vi "Main.vi"(8 "error in":errorcluster, 11 "Main View in":refnum<class "Main View.lvclass">) -> (0 "error out":errorcluster, 3 "Main View out":refnum<class "Main View.lvclass">)   [LabVIEW 2018, in "Main View.lvclass"]
doc: "The Queued Message Handler of a Worker."
uses:
  Main View.lvclass
  D:/Program Files (x86)/National Instruments/LabVIEW 2018/vi.lib/addons/_Workers/Library/Classes/Worker/Worker.lvclass
  Menu Button.ctl
  Main View.lvclass/Main View.ctl
  <vilib>/addons/_Workers/Library/Classes/Worker/Worker.lvclass/Worker.ctl
  Aging View/Aging View.lvclass
  Query Data/Query Data.lvclass
  About View/About View.lvclass
  Settings View/Settings View.lvclass
  <vilib>/addons/_Workers/Library/Classes/Message/Enqueue Message to Queue.vi
  <vilib>/addons/_Workers/Library/Classes/Message/Enqueue Message to Self v2.vi
  Acquire Data/Acquire Data.lvclass
  Save Data/Save Data.lvclass
  Initialization Data.ctl
  <vilib>/addons/_Workers/Library/Classes/Worker/Worker.lvclass
  <vilib>/addons/_Workers/Library/Classes/Message/Message.lvclass
  D:/Program Files (x86)/National Instruments/LabVIEW 2018/vi.lib/addons/_Workers/Library/Classes/Workers Object/Workers Object.lvclass
panel:
  in  "Menu Button":T1
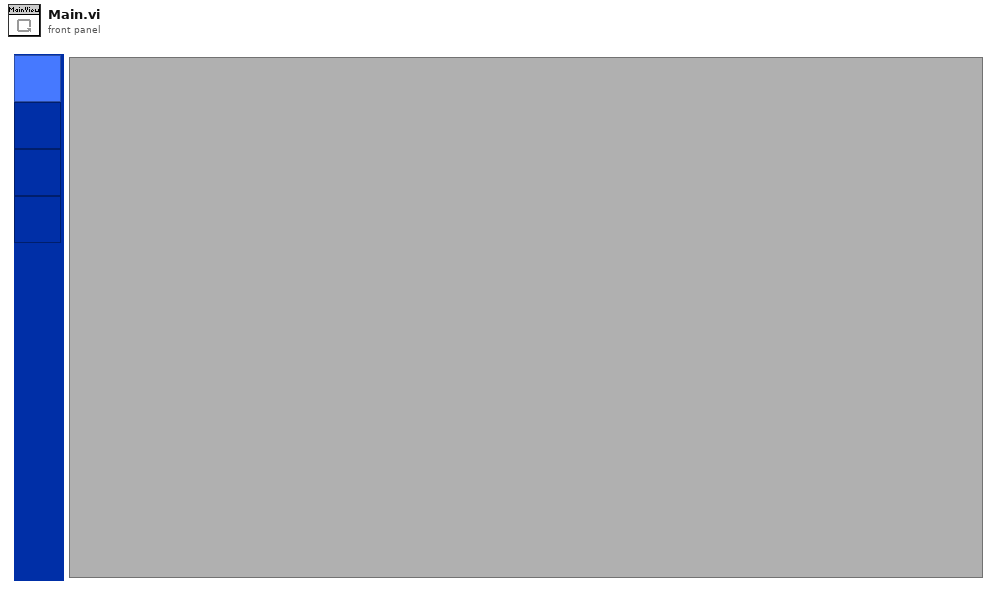
[diagram p1: front panel]
types:
  T1 = typedef "Main View.lvclass/Menu Button.ctl" = enum32{"Settings Button", "Aging Button", "Query Button", "Help Button"}
  T2 = typedef "Main View.lvclass/Initialization Data.ctl" = cluster{}
  T3 = typedef "Workers.lvlib/Case Label.ctl" = string
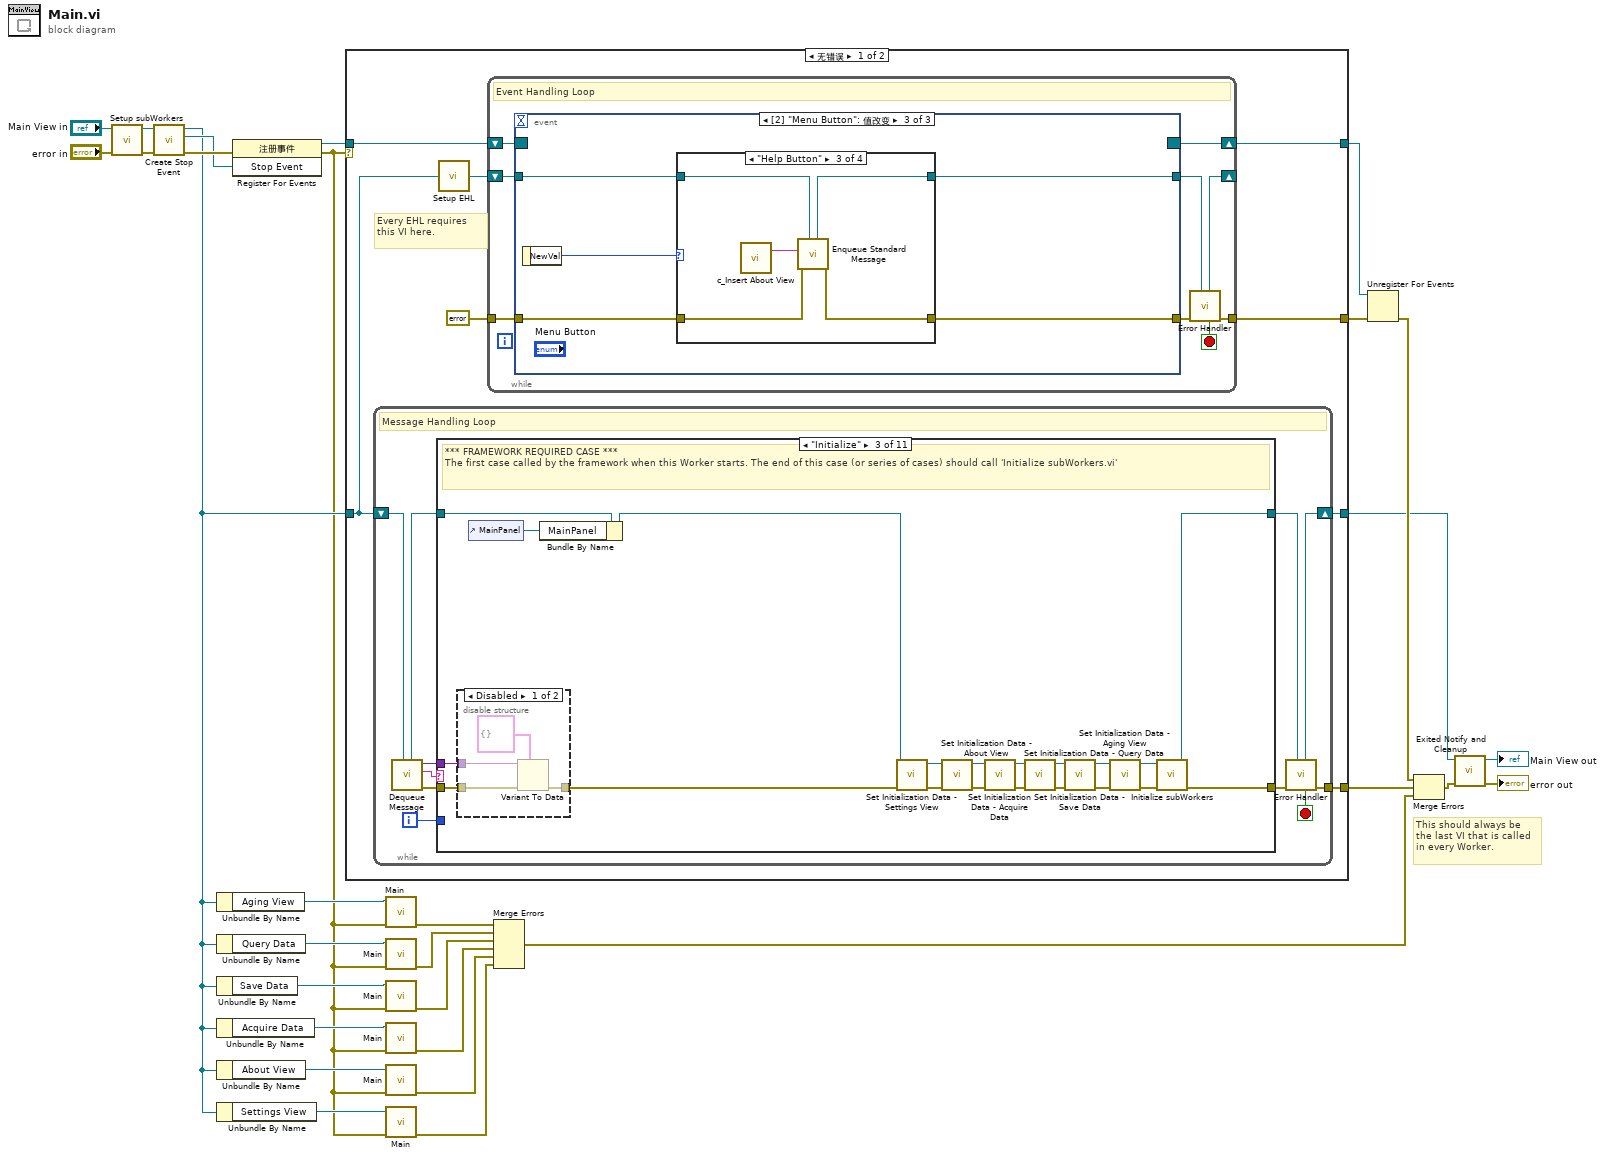
[diagram p0: block diagram]
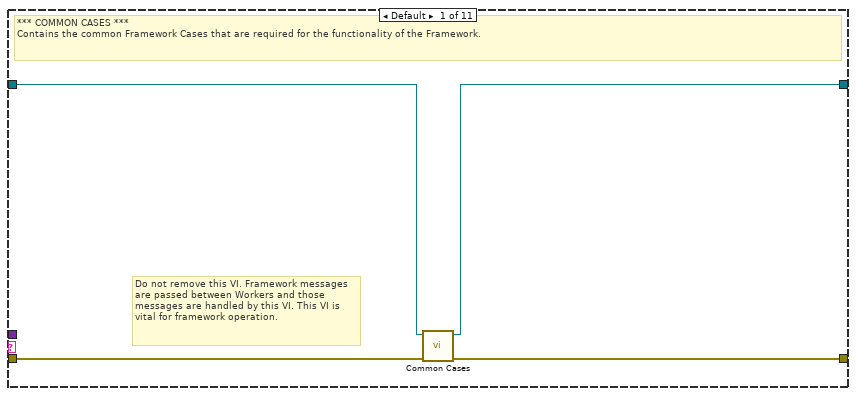
[diagram p2: hidden frame]
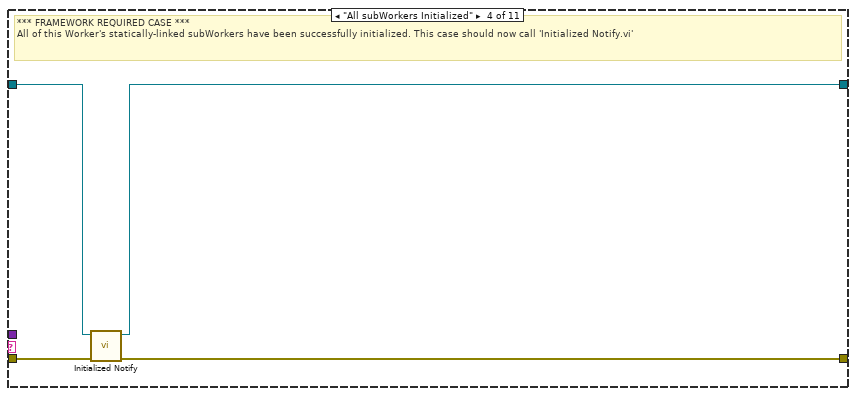
[diagram p5: hidden frame]
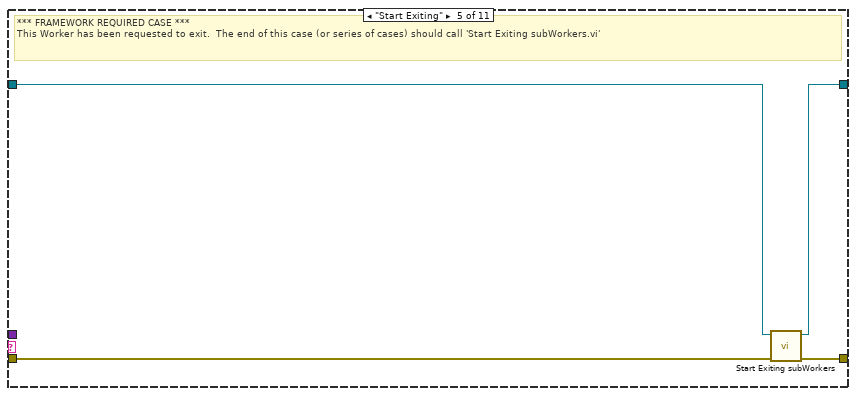
[diagram p6: hidden frame]
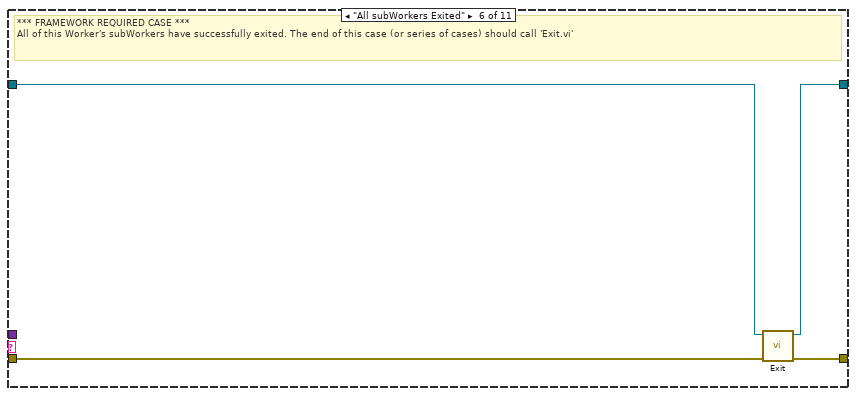
[diagram p7: hidden frame]
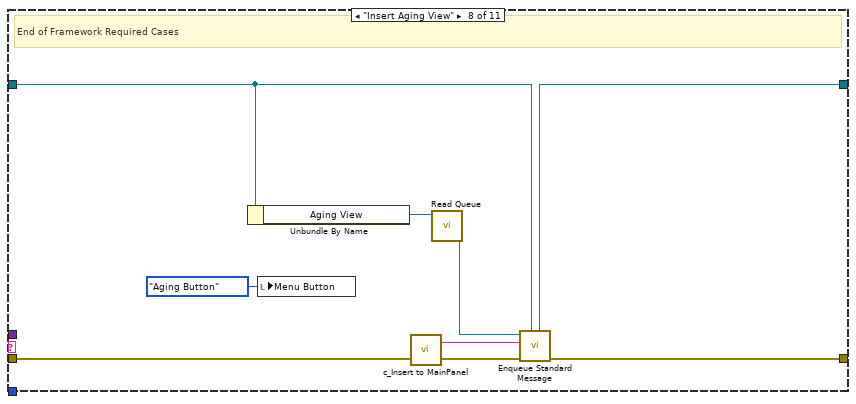
[diagram p9: hidden frame]
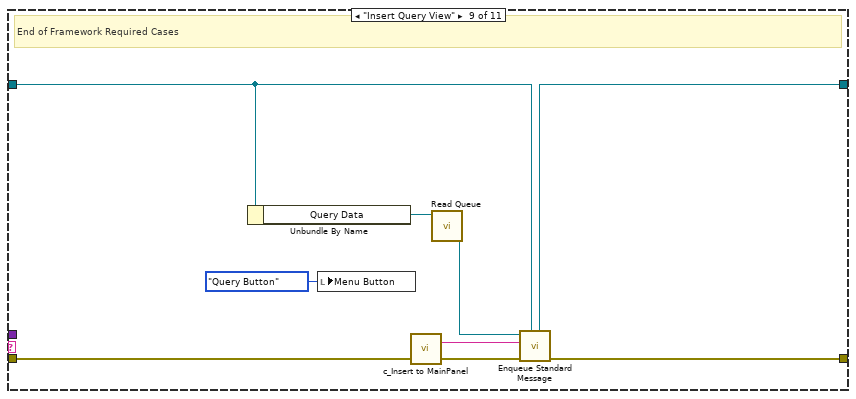
[diagram p10: hidden frame]
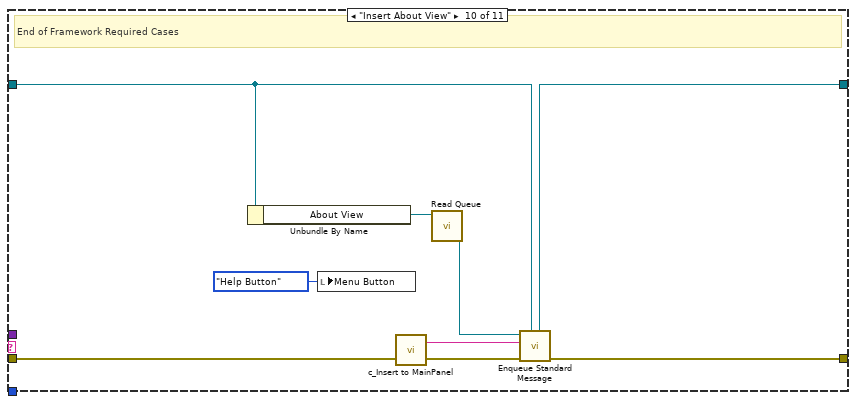
[diagram p11: hidden frame]
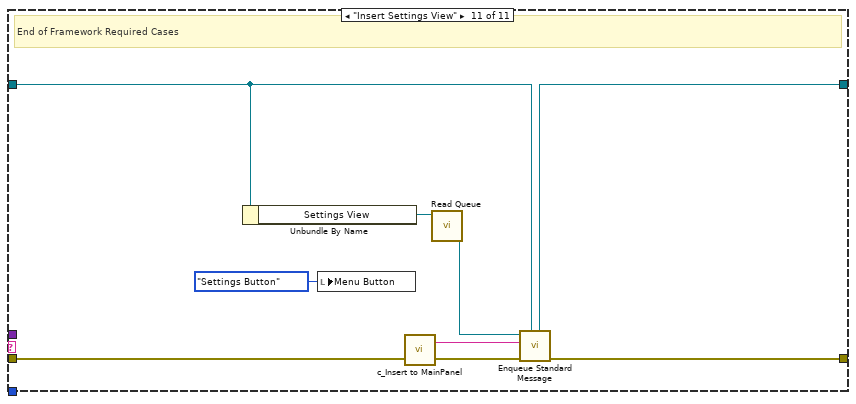
[diagram p12: hidden frame]
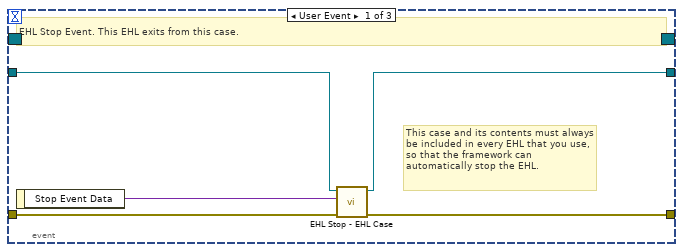
[diagram p13: hidden frame]
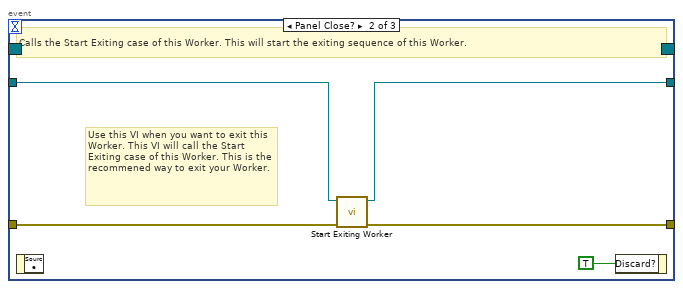
[diagram p14: hidden frame]
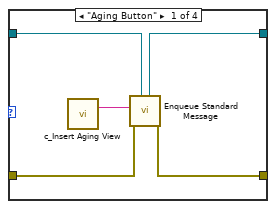
[diagram p15: hidden frame]
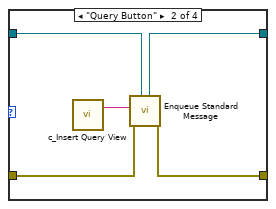
[diagram p16: hidden frame]
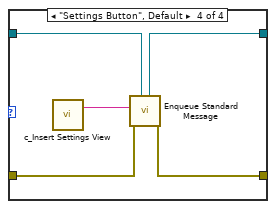
[diagram p17: hidden frame]
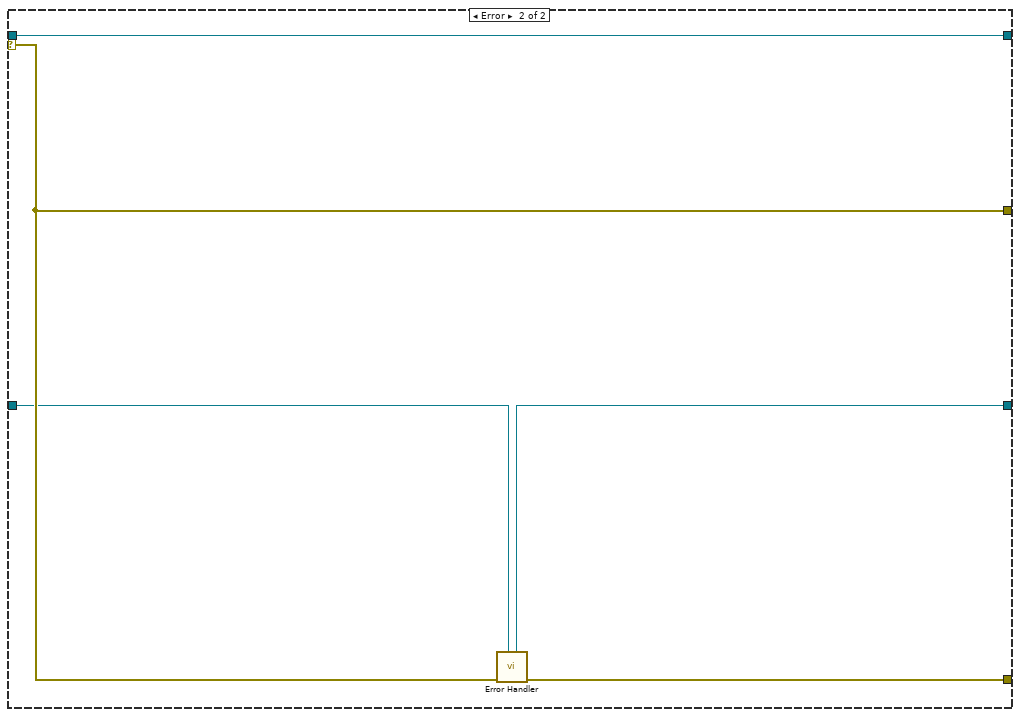
[diagram p18: hidden frame]
diagram:
  # "This should always be the last VI that is called in every Worker."
  n1 = call "Setup subWorkers.vi"("error in"="error in", "Main View in"="Main View in") -> ("error out"=w17:errorcluster, "Main View out"=w15:refnum<class "Main View.lvclass">)  [unwired: 8 in]
  n2 = call-dynamic "Create Stop Event.vi"("error in"=w17, "Worker"=w15) -> ("error out"=w25:errorcluster, "Stop Event"=w22:refnum<user-event>, "Worker out"=w19:refnum<class "Main View.lvclass">)  [unwired: 7 in]
  n3 = Unbundle By Name(w19) -> ("Aging View"=w13:refnum<class "Aging View.lvclass">)
  n4 = Unbundle By Name(w19) -> ("Query Data"=w11:refnum<class "Query Data.lvclass">)
  n5 = Unbundle By Name(w19) -> ("Save Data"=w9:refnum<class "Save Data.lvclass">)
  n6 = Unbundle By Name(w19) -> ("Acquire Data"=w7:refnum<class "Acquire Data.lvclass">)
  n7 = Unbundle By Name(w19) -> ("About View"=w5:refnum<class "About View.lvclass">)
  n8 = Unbundle By Name(w19) -> ("Settings View"=w3:refnum<class "Settings View.lvclass">)
  n9 = register-events(error in=w25, w22) -> (reference out=w24:refnum<event-registration>, error out=w1:errorcluster)  [unwired: 1 in]
  n10 = case shown="无错误" w1 {
    tunnel: w19 -> [w33 w172]
    tunnel: [w31 w173] -> w23
    tunnel: w24 -> [w38 w174]
    tunnel: [w35 w175] -> w29
    tunnel: [w37 w174] -> w28
    tunnel: [w32 w171] -> w26
    selector: w1 -> [_ w175]
    frame No Error {
      # "Every EHL requires\nthis VI here."
      n11 = while {
        shift-right: [w47] -> w32
        shift-left: w33 -> [w49]
        tunnel: [w48] -> w31
        i -> [w39]
        stop <- w40 stop-if-true
        # "Message Handling Loop"
        n12 = call-dynamic "Dequeue Message.vi"("Worker"=w49) -> ("error out"=w46:errorcluster, "Case out"=w41:string, "Data out"=w42:variant, "Worker out"=w44:refnum<class "Main View.lvclass">)  [unwired: 6 in, 1 out]
        n13 = case "Worker MHL Case Structure (DO NOT CHANGE LABEL NAME)" shown="\"Initialize\"" w41 {
          tunnel: w46 -> [w53 w54 w75 w83 w85 w92 w93 w99 w108 w116 w124]
          tunnel: [w52 w54 w57 w81 w88 w91 w93 w98 w107 w115 w123] -> w45
          tunnel: w44 -> [w51 w55 w73 w84 w86 w90 w94 w96 w105 w113 w121]
          tunnel: [w50 w55 w58 w82 w87 w89 w94 w97 w106 w114 w122] -> w43
          tunnel: w42 -> [_ _ w74 _ _ _ _ _ _ _ _]
          tunnel: w39 -> [_ _ _ _ _ _ _ _ _ _ _]
          frame Default {
            # "Do not remove this VI. Framework messages are passed between Workers and those messages are handled by this VI. This VI is vital for framework operation."
            # "*** COMMON CASES ***\nContains the common Framework Cases that are required for the functionality of the Framework."
            n14 = call-dynamic "Common Cases.vi"("error in"=w53, "Worker in"=w51) -> ("error out"=w52:errorcluster, "Worker out"=w50:refnum<class "Main View.lvclass">)  [unwired: 8 in]
          }
          frame "------ FRAMEWORK REQUIRED CASES ------" {
            # "Start of Framework Required Cases"
          }
          frame "Initialize" {
            # "*** FRAMEWORK REQUIRED CASE ***\nThe first case called by the framework when this Worker starts. The end of this case (or series of cases) should call 'Initialize subWorkers.vi'"
            n15 = disable-structure shown="Disabled" {
              disable-tunnel: w75 -> [w79 w80]
              disable-tunnel: [w78 w80] -> w56
              disable-tunnel: w74 -> [w77 _]
              frame Disabled {
                n16 = Variant To Data(error in=w79, type=T2 {} ("Initialization Data"), Variant=w77) -> (error out=w78:errorcluster)  [unwired: 1 out]
              }
              frame Enabled {
              }
            }
            n17 = control-ref of="MainPanel"() -> (w72:refnum<vi>)
            n18 = Bundle By Name(cluster=w73, "MainPanel"=w72) -> (w61:refnum<class "Main View.lvclass">)
            n19 = call "Set Initialization Data - Settings View.vi"("error in"=w56, "Main View in"=w61) -> ("error out"=w63:errorcluster, "Main View out"=w62:refnum<class "Main View.lvclass">)  [unwired: 8 in]
            n20 = call "Set Initialization Data - About View.vi"("error in"=w63, "Main View in"=w62) -> ("error out"=w64:errorcluster, "Main View out"=w65:refnum<class "Main View.lvclass">)  [unwired: 8 in]
            n21 = call "Set Initialization Data - Acquire Data.vi"("error in"=w64, "Main View in"=w65) -> ("error out"=w70:errorcluster, "Main View out"=w71:refnum<class "Main View.lvclass">)  [unwired: 8 in]
            n22 = call "Set Initialization Data - Query Data.vi"("error in"=w70, "Main View in"=w71) -> ("error out"=w68:errorcluster, "Main View out"=w69:refnum<class "Main View.lvclass">)  [unwired: 8 in]
            n23 = call "Set Initialization Data - Save Data.vi"("error in"=w68, "Main View in"=w69) -> ("error out"=w67:errorcluster, "Main View out"=w66:refnum<class "Main View.lvclass">)  [unwired: 8 in]
            n24 = call "Set Initialization Data - Aging View.vi"("error in"=w67, "Main View in"=w66) -> ("error out"=w59:errorcluster, "Main View out"=w60:refnum<class "Main View.lvclass">)  [unwired: 8 in]
            n25 = call-dynamic "Initialize subWorkers.vi"("error in"=w59, "Worker"=w60) -> ("error out"=w57:errorcluster, "dup Worker out"=w58:refnum<class "Main View.lvclass">)  [unwired: 8 in]
          }
          frame "All subWorkers Initialized" {
            # "*** FRAMEWORK REQUIRED CASE ***\nAll of this Worker's statically-linked subWorkers have been successfully initialized. This case should now call 'Initialized Notify.vi'"
            n26 = call-dynamic "Initialized Notify.vi"("error in"=w83, "Worker"=w84) -> ("error out"=w81:errorcluster, "dup Worker out"=w82:refnum<class "Main View.lvclass">)  [unwired: 8 in]
          }
          frame "Start Exiting" {
            # "*** FRAMEWORK REQUIRED CASE ***\nThis Worker has been requested to exit.  The end of this case (or series of cases) should call 'Start Exiting subWorkers.vi'"
            n27 = call-dynamic "Start Exiting subWorkers.vi"("error_in"=w85, "Worker"=w86) -> ("error out"=w88:errorcluster, "dup Worker out"=w87:refnum<class "Main View.lvclass">)  [unwired: 8 in]
          }
          frame "All subWorkers Exited" {
            # "*** FRAMEWORK REQUIRED CASE ***\nAll of this Worker's subWorkers have successfully exited. The end of this case (or series of cases) should call 'Exit.vi'"
            n28 = call-dynamic "Exit.vi"("error_in"=w92, "Worker"=w90) -> ("error out"=w91:errorcluster, "dup Worker out"=w89:refnum<class "Main View.lvclass">)  [unwired: 8 in]
          }
          frame "-----------------------------------------------" {
            # "End of Framework Required Cases"
          }
          frame "Insert Aging View" {
            # "End of Framework Required Cases"
            n29 = Unbundle By Name(w96) -> ("Aging View"=w102:refnum<class "Aging View.lvclass">)
            n30 = local write "Menu Button"(Menu_Button."Aging Button" ("Menu Button")) -> ()
            n31 = call "c_Insert to MainPanel.vi"() -> ("Case Label"=w100:T3)  [unwired: 1 in]
            n32 = call <vilib>:"Read Queue.vi"("Worker"=w102) -> ("Message Queue out"=w101:refnum<class "Message Queue.lvclass">)  [unwired: 9 in, 1 out]
            n33 = call-poly <vilib>:"Enqueue Standard Message.vi"("Worker"=w96, "error in"=w99, "Case Label"=w100, "Message Queue"=w101) -> ("error out"=w98:errorcluster, "dup Worker out"=w97:refnum<class "Main View.lvclass">)  [unwired: 5 in, 1 out]
          }
          frame "Insert Query View" {
            # "End of Framework Required Cases"
            n34 = Unbundle By Name(w105) -> ("Query Data"=w110:refnum<class "Query Data.lvclass">)
            n35 = local write "Menu Button"(Menu_Button."Query Button" ("Menu Button")) -> ()
            n36 = call "c_Insert to MainPanel.vi"() -> ("Case Label"=w104:T3)  [unwired: 1 in]
            n37 = call <vilib>:"Read Queue.vi"("Worker"=w110) -> ("Message Queue out"=w109:refnum<class "Message Queue.lvclass">)  [unwired: 9 in, 1 out]
            n38 = call-poly <vilib>:"Enqueue Standard Message.vi"("Worker"=w105, "error in"=w108, "Case Label"=w104, "Message Queue"=w109) -> ("error out"=w107:errorcluster, "dup Worker out"=w106:refnum<class "Main View.lvclass">)  [unwired: 5 in, 1 out]
          }
          frame "Insert About View" {
            # "End of Framework Required Cases"
            n39 = Unbundle By Name(w113) -> ("About View"=w118:refnum<class "About View.lvclass">)
            n40 = local write "Menu Button"(Menu_Button."Help Button" ("Menu Button")) -> ()
            n41 = call "c_Insert to MainPanel.vi"() -> ("Case Label"=w111:T3)  [unwired: 1 in]
            n42 = call <vilib>:"Read Queue.vi"("Worker"=w118) -> ("Message Queue out"=w117:refnum<class "Message Queue.lvclass">)  [unwired: 9 in, 1 out]
            n43 = call-poly <vilib>:"Enqueue Standard Message.vi"("Worker"=w113, "error in"=w116, "Case Label"=w111, "Message Queue"=w117) -> ("error out"=w115:errorcluster, "dup Worker out"=w114:refnum<class "Main View.lvclass">)  [unwired: 5 in, 1 out]
          }
          frame "Insert Settings View" {
            # "End of Framework Required Cases"
            n44 = Unbundle By Name(w121) -> ("Settings View"=w126:refnum<class "Settings View.lvclass">)
            n45 = local write "Menu Button"(Menu_Button."Settings Button" ("Menu Button")) -> ()
            n46 = call "c_Insert to MainPanel.vi"() -> ("Case Label"=w119:T3)  [unwired: 1 in]
            n47 = call <vilib>:"Read Queue.vi"("Worker"=w126) -> ("Message Queue out"=w125:refnum<class "Message Queue.lvclass">)  [unwired: 9 in, 1 out]
            n48 = call-poly <vilib>:"Enqueue Standard Message.vi"("Worker"=w121, "error in"=w124, "Case Label"=w119, "Message Queue"=w125) -> ("error out"=w123:errorcluster, "dup Worker out"=w122:refnum<class "Main View.lvclass">)  [unwired: 5 in, 1 out]
          }
        }
        n49 = call-dynamic "Error Handler.vi"("Worker"=w43, "error_in"=w45) -> ("error out"=w48:errorcluster, "Stop Loop"=w40:bool, "Worker out"=w47:refnum<class "Main View.lvclass">)  [unwired: 7 in]
      }
      n50 = call-dynamic "Setup EHL.vi"("Worker"=w33) -> ("Worker out"=w34:refnum<class "Main View.lvclass">)  [unwired: 14 in]
      n51 = while "Event Handling Loop" {
        shift-right: [w135] -> w37
        shift-left: w38 -> [w134]
        tunnel: [w130] -> w35
        tunnel: errorcluster {"status"=FALSE, "code"=0, "source"=""} ("error constant") -> [w132]
        shift-right: [w128] -> _
        shift-left: w34 -> [w133]
        stop <- w127 stop-if-true
        # "Event Handling Loop"
        n52 = event shown="[2] \"Menu Button\": 值改变" {
          selector: w134 -> [_ _ _]
          dyn-events: [_ _ _] -> w135
          timeout: _ -> [_ _ _]
          tunnel: [w139 w144 w146] -> w131
          tunnel: w132 -> [w140 w143 w147]
          tunnel: w133 -> [w138 w142 w149]
          tunnel: [w137 w141 w148] -> w129
          event User Event {
            # "This case and its contents must always be included in every EHL that you use, so that the framework can automatically stop the EHL."
            # "EHL Stop Event. This EHL exits from this case."
            n53 = event-data() -> ("Stop Event Data"=w136:variant)  [unwired: 1 in]
            n54 = call <vilib>:"EHL Stop - EHL Case.vi"("error in"=w140, "Stop Event Data"=w136, "Worker"=w138) -> ("error out"=w139:errorcluster, "Worker out"=w137:refnum<class "Main View.lvclass">)  [unwired: 7 in]
          }
          event Panel Close? {
            # "Use this VI when you want to exit this Worker. This VI will call the Start Exiting case of this Worker. This is the recommened way to exit your Worker."
            # "Calls the Start Exiting case of this Worker. This will start the exiting sequence of this Worker."
            n55 = event-data() -> ()  [unwired: 1 in, 1 out]
            n56 = call-dynamic "Start Exiting Worker.vi"("error in"=w143, "Worker"=w142) -> ("error out"=w144:errorcluster, "dup Worker out"=w141:refnum<class "Main View.lvclass">)  [unwired: 8 in]
            n57 = event-data ("Event Filter Node")("Discard?"=TRUE) -> ()  [unwired: 1 in, 1 out]
          }
          event Value Change {
            n58 = event-data() -> ("NewVal"=w150:T1)  [unwired: 1 in]
            n59 = case shown="\"Help Button\"" w150 {
              tunnel: w149 -> [w155 w160 w165 w170]
              tunnel: [w154 w159 w164 w169] -> w148
              tunnel: w147 -> [w153 w158 w163 w168]
              tunnel: [w152 w157 w162 w167] -> w146
              frame "Aging Button" {
                n60 = call "c_Insert Aging View.vi"() -> ("Case Label"=w151:T3)  [unwired: 1 in]
                n61 = call-poly <vilib>:"Enqueue Standard Message.vi"("Worker"=w155, "error in"=w153, "Case Label"=w151) -> ("error out"=w152:errorcluster, "dup Worker out"=w154:refnum<class "Main View.lvclass">)  [unwired: 7 in]
              }
              frame "Query Button" {
                n62 = call "c_Insert Query View.vi"() -> ("Case Label"=w156:T3)  [unwired: 1 in]
                n63 = call-poly <vilib>:"Enqueue Standard Message.vi"("Worker"=w160, "error in"=w158, "Case Label"=w156) -> ("error out"=w157:errorcluster, "dup Worker out"=w159:refnum<class "Main View.lvclass">)  [unwired: 7 in]
              }
              frame "Help Button" {
                n64 = call "c_Insert About View.vi"() -> ("Case Label"=w161:T3)  [unwired: 1 in]
                n65 = call-poly <vilib>:"Enqueue Standard Message.vi"("Worker"=w165, "error in"=w163, "Case Label"=w161) -> ("error out"=w162:errorcluster, "dup Worker out"=w164:refnum<class "Main View.lvclass">)  [unwired: 7 in]
              }
              frame "Settings Button", Default {
                n66 = call "c_Insert Settings View.vi"() -> ("Case Label"=w166:T3)  [unwired: 1 in]
                n67 = call-poly <vilib>:"Enqueue Standard Message.vi"("Worker"=w170, "error in"=w168, "Case Label"=w166) -> ("error out"=w167:errorcluster, "dup Worker out"=w169:refnum<class "Main View.lvclass">)  [unwired: 7 in]
              }
            }
          }
        }
        n68 = call-dynamic "Error Handler.vi"("Worker"=w129, "error_in"=w131) -> ("error out"=w130:errorcluster, "Stop Loop"=w127:bool, "Worker out"=w128:refnum<class "Main View.lvclass">)  [unwired: 7 in]
      }
    }
    frame Error {
      n69 = call-dynamic "Error Handler.vi"("Worker"=w172, "error_in"=w175) -> ("error out"=w173:errorcluster, "Worker out"=w171:refnum<class "Main View.lvclass">)  [unwired: 7 in, 1 out]
    }
  }
  n70 = call-dynamic "Main.vi"("error in"=w1, "Aging View in"=w13) -> ("error out"=w14:errorcluster)  [unwired: 8 in, 1 out]
  n71 = call-dynamic "Main.vi"("error in"=w1, "Query Data in"=w11) -> ("error out"=w12:errorcluster)  [unwired: 8 in, 1 out]
  n72 = call-dynamic "Main.vi"("error in"=w1, "Save Data in"=w9) -> ("error out"=w10:errorcluster)  [unwired: 8 in, 1 out]
  n73 = call-dynamic "Main.vi"("error in"=w1, "Acquire Data in"=w7) -> ("error out"=w8:errorcluster)  [unwired: 8 in, 1 out]
  n74 = call-dynamic "Main.vi"("error in"=w1, "About View in"=w5) -> ("error out"=w6:errorcluster)  [unwired: 8 in, 1 out]
  n75 = call-dynamic "Main.vi"("error in"=w1, "Settings View in"=w3) -> ("error out"=w4:errorcluster)  [unwired: 8 in, 1 out]
  n76 = Merge Errors(w14, w12, w10, w8, w6, w4) -> (w2:errorcluster)
  n77 = Unregister For Events(event registration refnum=w28, error in=w29) -> (error out=w30:errorcluster)
  n78 = Merge Errors(w30, w23, w2) -> (w27:errorcluster)
  n79 = call-dynamic "Exited Notify and Cleanup.vi"("error_in"=w27, "Worker"=w26) -> ("error out"=→"error out":errorcluster, "dup Worker out"=→"Main View out":refnum<class "Main View.lvclass">)  [unwired: 8 in]
